vi "rot2.vi"(4 "error in":errorcluster, 5 "Bool Refnum":refnum<vi>, 7 "Arr Refnum":refnum<vi>) -> (1 "too many ers":bool)   [LabVIEW 2010]
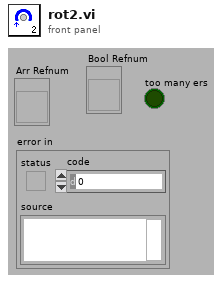
[diagram p1: front panel]
types:
  T1 = cluster{"seconds since 1Jan1904":timestamp, "source":string}
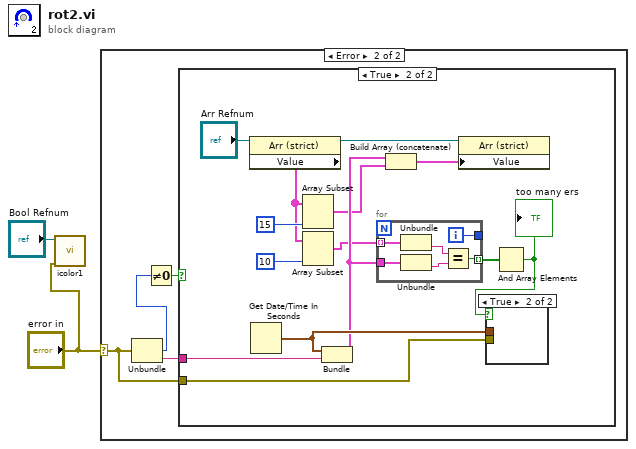
[diagram p0: block diagram]
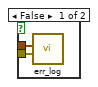
[diagram p4: hidden frame]
diagram:
  n1 = call "icolor1.vi"("error in (no error)"="error in", "Bool Refnum"="Bool Refnum") -> ()  [unwired: 6 in]
  n2 = case shown="Error" "error in" {
    selector: "error in" -> [_ w3]
    frame No Error {
    }
    frame Error {
      n3 = Unbundle(w3) -> ("code"=w4:i32, "source"=w6:string)  [unwired: 1 out]
      n4 = Not Equal To 0?(x=w4) -> (x != 0?=w5:bool)
      n5 = case shown="True" w5 {
        tunnel: w6 -> [_ w20]
        tunnel: w3 -> [_ w15]
        frame False {
        }
        frame True {
          n6 = property on="Property Node" class="Arr (strict)"(reference="Arr Refnum") -> (reference out=w18:refnum<vi>, "Value"=w9:cluster{"time stamp":timestamp, "t0":string}[])  [unwired: 1 in, 1 out]
          n7 = Get Date/Time In Seconds() -> (seconds since 1Jan1904=w16:timestamp)
          n8 = Array Subset(array=w9, length=15) -> (w11:cluster{"time stamp":timestamp, "t0":string}[])  [unwired: 1 in]
          n9 = Array Subset(array=w9, length=10 ("y")) -> (w8:cluster{"time stamp":timestamp, "t0":string}[])  [unwired: 1 in]
          n10 = Bundle("seconds since 1Jan1904"=w16, "source"=w20) -> (w14:T1)  [unwired: 1 in]
          n11 = for {
            tunnel: w8 -> [w28] mode=indexing
            tunnel: w14 -> [w27]
            tunnel: [w24] -> w13 mode=indexing
            tunnel: [w23] -> _
            i -> [w23]
            n12 = Unbundle(w28) -> ("t0"=w25:string)  [unwired: 1 out]
            n13 = Unbundle(w27) -> ("source"=w26:string)  [unwired: 1 out]
            n14 = Equal?(x=w25, y=w26) -> (x = y?=w24:bool)
          }
          n15 = Build Array (concatenate)(w14, w11) -> (w12:cluster{"time stamp":timestamp, "t0":string}[])
          n16 = property on="Property Node" class="Arr (strict)"(reference=w18, "Value"=w12) -> ()  [unwired: 1 in, 2 out]
          n17 = And Array Elements(Boolean array=w13) -> (logical AND=w7:bool)
          "too many ers" <- w7
          n18 = case shown="True" w7 {
            tunnel: w16 -> [w22 _]
            tunnel: w15 -> [w21 _]
            frame False {
              n19 = call "err_log.vi"("error In"=w21, "time stamp"=w22) -> ()  [unwired: 4 in, 2 out]
            }
            frame True {
            }
          }
        }
      }
    }
  }
